vi "Is string in string.vi"(8 "error in (no error)":errorcluster, 10 "Search for string":string, 11 "String buffer":string) -> (0 "error out":errorcluster, 3 "In string?":bool)   [LabVIEW 2024]
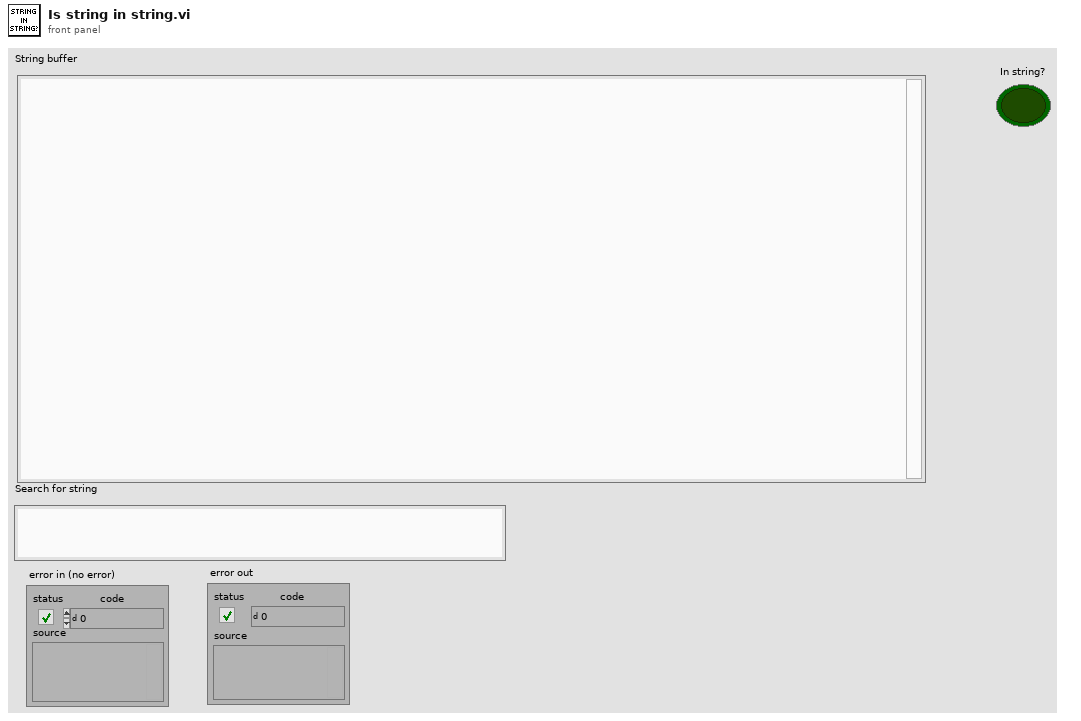
[diagram p1: front panel]
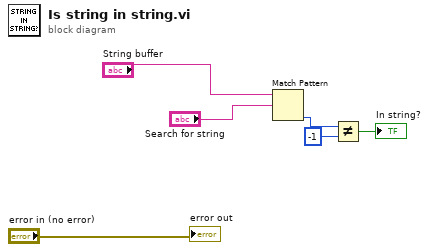
[diagram p0: block diagram]
diagram:
  n1 = Match Pattern(string="String buffer", regular expression="Search for string") -> (offset past match=w5:i32)  [unwired: 1 in, 3 out]
  n2 = Not Equal?(x=w5, y=-1) -> (x != y?=→"In string?":bool)
  "error out" <- "error in (no error)"
